vi "Round.vi"(10 "Val":dbl, 11 "Step":dbl) -> (3 "Val'":dbl)   [LabVIEW 2018]
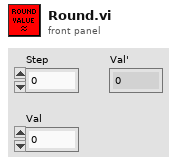
[diagram p1: front panel]
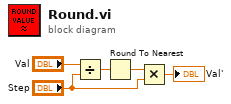
[diagram p0: block diagram]
diagram:
  n1 = Divide(x="Val", y="Step") -> (x/y=w4:dbl)
  n2 = Round To Nearest(number=w4) -> (nearest integer value=w3:dbl)
  n3 = Multiply(x=w3, y="Step") -> (x*y=→"Val'":dbl)
